vi "恢复参数.vi"(8 "仪器公式":T2(array[cluster]), 9 "量程参数":T3(array[cluster]), 10 "试剂容量参数":T4, 11 "外设参数":cluster{"仪器版本":T1, "error out":errorcluster}) -> (3 "恢复结果":string)   [LabVIEW 2016, in "斯坦道总磷总氮.lvlib"]
uses:
  <vilib>/NI/Progress Bar/Progress Bar.lvlib
  <vilib>/Utility/config.llb/NI_LVConfig.lvlib
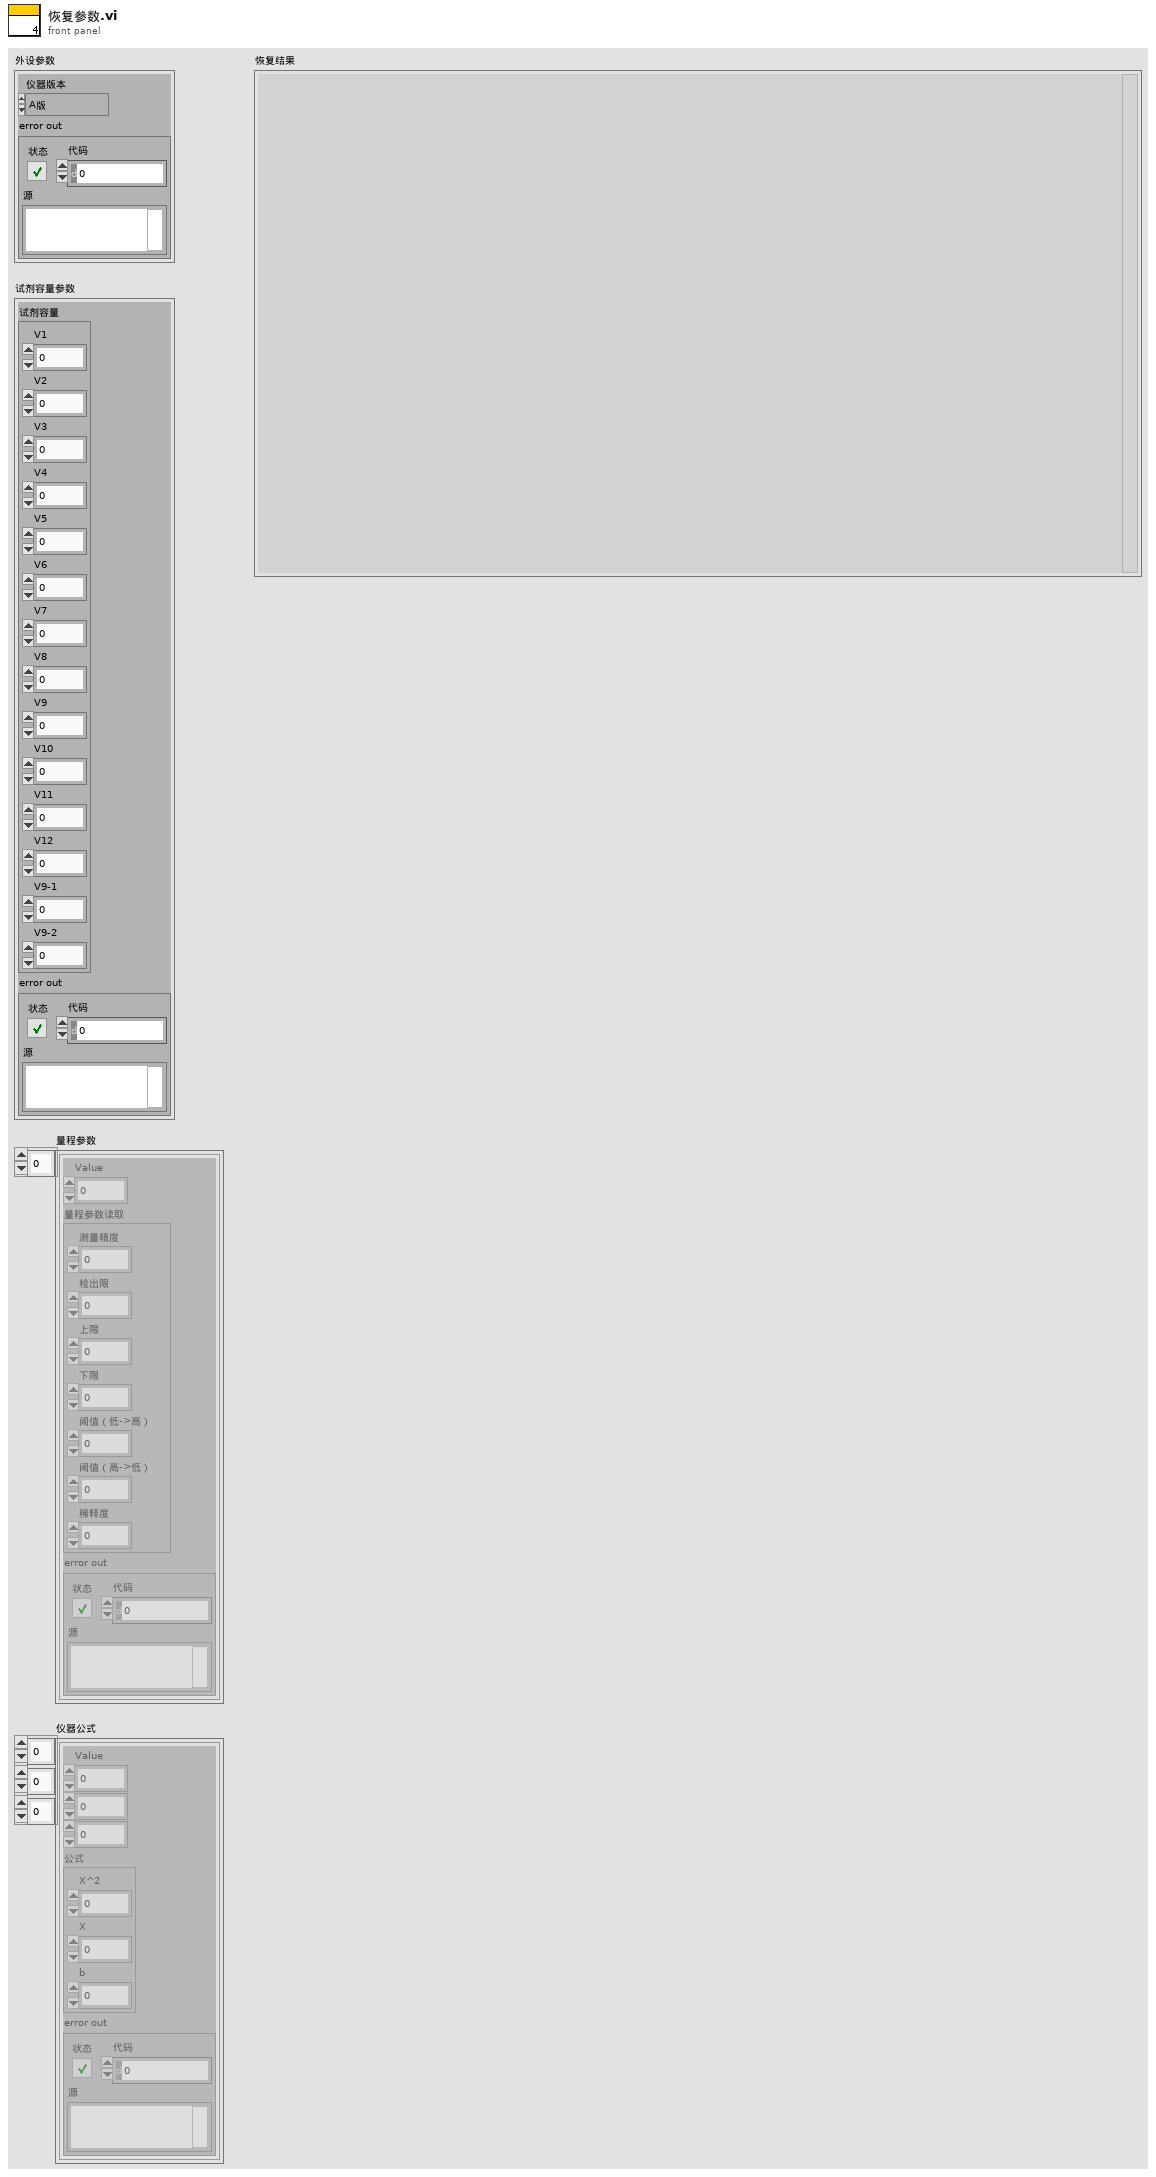
[diagram p1: front panel]
types:
  T1 = typedef "SingleStepTestV3.lvlib/SingleStepTestV3.lvclass/仪器版本.ctl" = enum16{"A版", "B版", "A1版"}
  T2 = cluster{"Value":u16, i32, i32, "公式":cluster{"X^2":dbl, "X":dbl, "b":dbl}, "error out":errorcluster}[][][]
  T3 = cluster{"Value":u16, "量程参数读取":cluster{"测量精度":u16, "检出限":dbl, "上限":dbl, "下限":dbl, "阈值（低->高）":dbl, "阈值（高->低）":dbl, "稀释度":dbl}, "error out":errorcluster}[]
  T4 = cluster{"试剂容量":cluster{"V1":sgl, "V2":sgl, "V3":sgl, "V4":sgl, "V5":sgl, "V6":sgl, "V7":sgl, "V8":sgl, "V9":sgl, "V10":sgl, "V11":sgl, "V12":sgl, "V9-1":sgl, "V9-2":sgl}, "error out":errorcluster}
  T5 = enum16{"恢复外设参数", "恢复试剂容量参数", "恢复量程参数", "恢复仪器公式", "结束"}
  T6 = typedef "NI_LVConfig.lvlib/Config Data RefNum.ctl" = refnum<k1>
  T7 = typedef "斯坦道总磷总氮.lvlib/V3 A版外设参数.ctl" = cluster{"泵类型":u8, "进样速度":u32, "出样速度":u32, "泵阀量":u8, "阀方向":u8, "光谱仪类型":u8, "光谱采样次数":u8, "氙灯次数":u8, "B":u16, "C":u16, "D":u16, "E":u16, "B_COD":u16, "C_COD":u16, "D_COD":u16, "E_COD":u16, "G":u16, "M":u16, "N":u16, "氨氮注射泵控温下限":sgl, "氨氮注射泵控温上限":sgl, "总氮注射泵控温下限":sgl, "总氮注射泵控温上限":sgl, "消解温度下限":sgl, "消解温度上限":sgl, "加热10s限值":sgl, "KP":sgl, "KI":sgl, "KD":sgl, "高温高压阀开阀温度":sgl, "总氮x公式0":u8, "总氮x公式1":sgl, "总氮x公式2":sgl, "总磷浊度稀释系数":sgl, "总磷浊度补偿权重1":sgl, "总磷浊度补偿权重2":sgl, "盐度系数":sgl, "氨氮补偿系数1":sgl, "氨氮补偿系数2":sgl}
  T8 = typedef "斯坦道总磷总氮.lvlib/V3 B版外设参数.ctl" = cluster{"泵类型":u8, "注射泵正常速度":u32, "注射泵慢速":u32, "阀型号":u8, "res":u8, "光谱仪类型":u8, "光谱采样次数":u8, "氙灯次数":u8, "B":u16, "C":u16, "D":u16, "E":u16, "B_COD":u16, "C_COD":u16, "D_COD":u16, "E_COD":u16, "G":u16, "M":u16, "N":u16, "降温下限":sgl, "降温上限":sgl, "恒温温度下限":sgl, "恒温温度上限":sgl, "消解温度下限":sgl, "消解温度上限":sgl, "加热10s限值":sgl, "KP":sgl, "KI":sgl, "KD":sgl, "高温高压阀开阀温度":sgl, "总氮x公式0":u8, "总氮x公式1":sgl, "总氮x公式2":sgl, "总磷浊度稀释系数":sgl, "总磷浊度补偿权重1":sgl, "总磷浊度补偿权重2":sgl, "盐度系数":sgl, "氨氮补偿系数1":sgl, "氨氮补偿系数2":sgl, "缺试剂传感器阈值":u16}
  T9 = typedef "斯坦道总磷总氮.lvlib/V3 A1版外设参数.ctl" = cluster{"泵类型":u8, "进样速度":u32, "出样速度":u32, "泵阀量":u8, "光谱仪类型":u8, "光谱采样次数":u8, "氙灯次数":u8, "B":u16, "C":u16, "D":u16, "E":u16, "B_COD":u16, "C_COD":u16, "D_COD":u16, "E_COD":u16, "G":u16, "M":u16, "N":u16, "氨氮注射泵控温下限":sgl, "氨氮注射泵控温上限":sgl, "总氮注射泵控温下限":sgl, "总氮注射泵控温上限":sgl, "消解温度下限":sgl, "消解温度上限":sgl, "加热10s限值":sgl, "高温高压阀开阀温度":sgl, "总氮x公式0":u8, "总氮x公式1":sgl, "总氮x公式2":sgl, "总磷浊度稀释系数":sgl, "总磷浊度补偿权重1":sgl, "总磷浊度补偿权重2":sgl, "盐度系数":sgl, "氨氮补偿系数1":sgl, "氨氮补偿系数2":sgl}
  T10 = cluster{"V1":sgl, "V2":sgl, "V3":sgl, "V4":sgl, "V5":sgl, "V6":sgl, "V7":sgl, "V8":sgl, "V9":sgl, "V10":sgl, "V11":sgl, "V12":sgl, "V9-1":sgl, "V9-2":sgl}
  T11 = cluster{"测量精度":u16, "检出限":dbl, "上限":dbl, "下限":dbl, "阈值（低->高）":dbl, "阈值（高->低）":dbl, "稀释度":dbl}
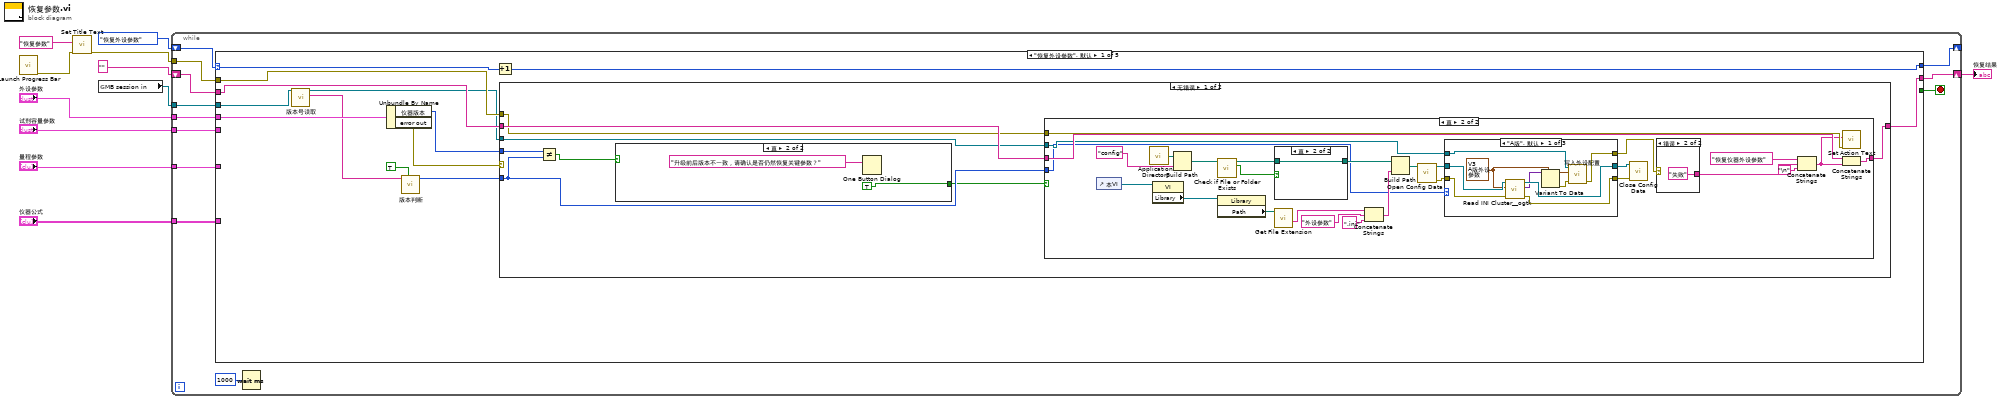
[diagram p0: block diagram]
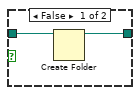
[diagram p3: hidden frame]
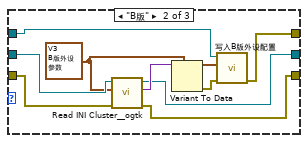
[diagram p4: hidden frame]
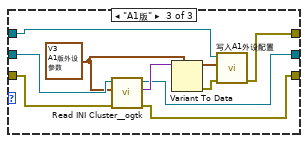
[diagram p5: hidden frame]
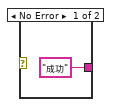
[diagram p6: hidden frame]
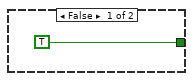
[diagram p7: hidden frame]
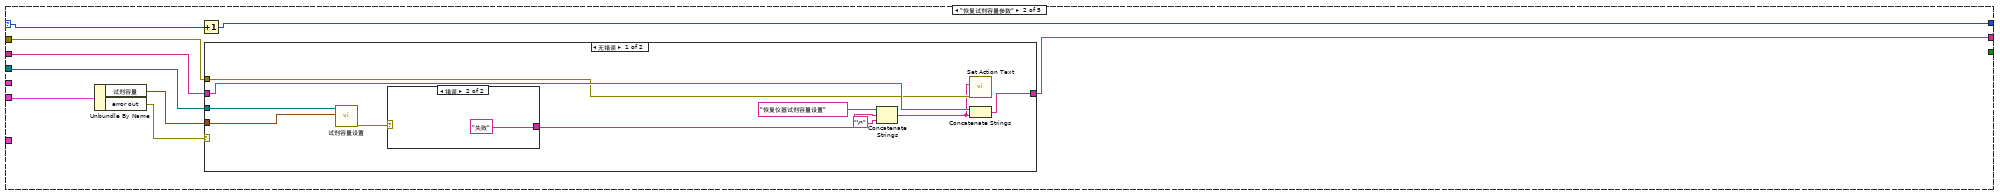
[diagram p9: hidden frame]
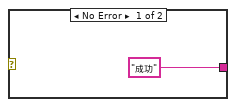
[diagram p10: hidden frame]
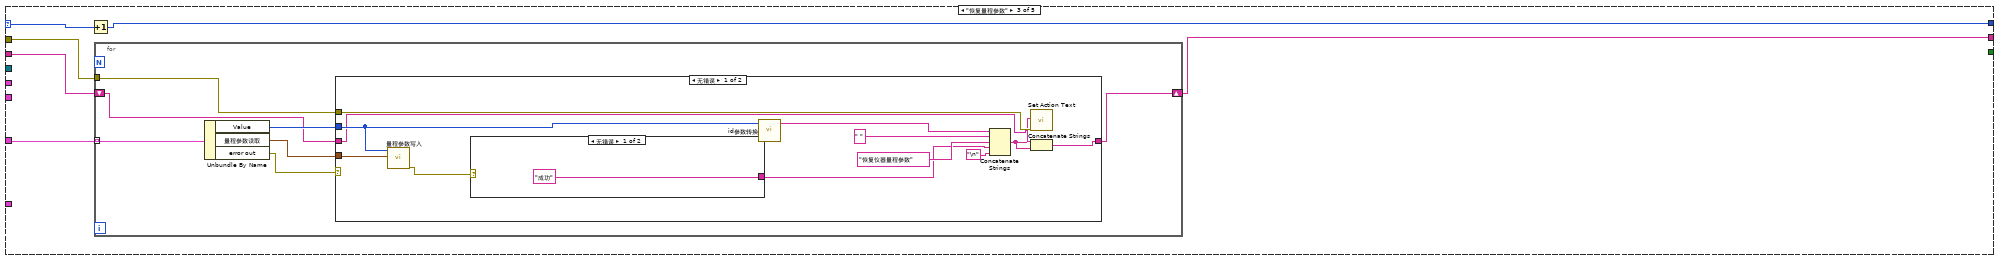
[diagram p12: hidden frame]
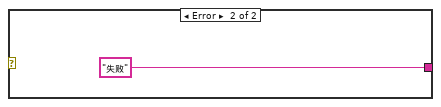
[diagram p13: hidden frame]
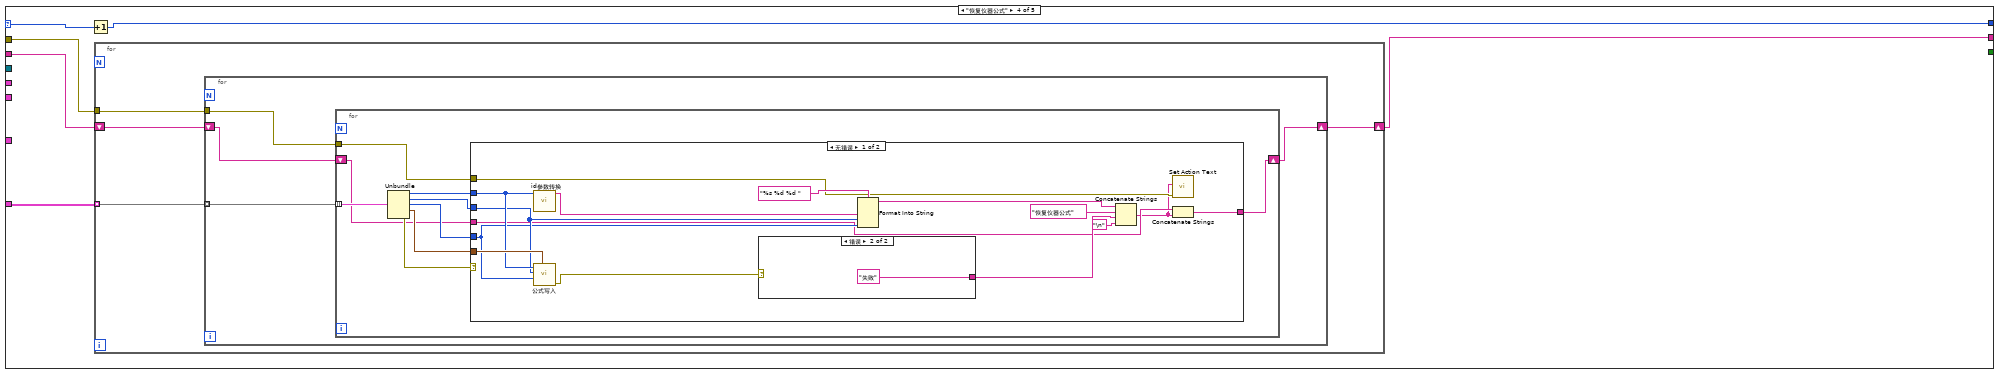
[diagram p15: hidden frame]
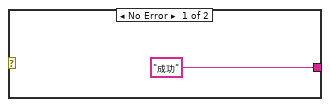
[diagram p16: hidden frame]
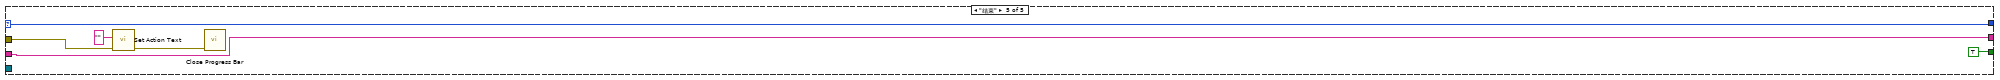
[diagram p18: hidden frame]
diagram:
  n1 = call <vilib>:"Launch Progress Bar.vi"() -> ("error out"=w4:errorcluster)  [unwired: 10 in, 1 out]
  n2 = call <vilib>:"Set Title Text.vi"("error in (no error)"=w4, "Installer Title"="恢复参数") -> ("error out"=w3:errorcluster)  [unwired: 9 in]
  n3 = global read "VAR总磷总氮全局变量.vi" "MB session in"() -> (w9:refnum<class "MB_Master.lvclass">)
  n4 = while {
    shift-right: [w22] -> _
    shift-left: T5."恢复外设参数" ("枚举") -> [w23]
    tunnel: "外设参数" -> [w21]
    shift-right: [w15] -> w5
    shift-left: "" -> [w20]
    tunnel: w9 -> [w19]
    tunnel: "试剂容量参数" -> [w18]
    tunnel: "量程参数" -> [w17]
    tunnel: "仪器公式" -> [w16]
    tunnel: w3 -> [w13]
    stop <- w14 stop-if-true
    n5 = case shown="\"恢复外设参数\", 默认" w23 {
      selector: w23 -> [w36 w121 w140 w168 w209]
      tunnel: [w35 w120 w139 w167 w209] -> w22
      tunnel: w21 -> [w30 _ _ _ _]
      tunnel: w20 -> [w33 w115 w137 w165 w208]
      tunnel: w19 -> [w28 w117 _ _ _]
      tunnel: w18 -> [_ w119 _ _ _]
      tunnel: w17 -> [_ _ w138 _ _]
      tunnel: w16 -> [_ _ _ w166 _]
      tunnel: [w32 w114 w136 w164 w208] -> w15
      tunnel: [_ _ _ _ TRUE] -> w14
      tunnel: w13 -> [w31 w113 w135 w163 w206]
      frame "恢复外设参数", Default {
        n6 = call "版本号读取.vi"("MB session in"=w28) -> ("固件版本号"=w26:string, "MB session out"=w27:refnum<class "MB_Master.lvclass">)  [unwired: 8 in, 1 out]
        n7 = Unbundle By Name(w30) -> ("仪器版本"=w24:T1, "error out"=w34:errorcluster)
        n8 = call "版本判断.vi"("Extern"=TRUE, "固件版本号"=w26) -> ("仪器版本"=w29:T1)  [unwired: 9 in]
        n9 = Increment(x=w36) -> (x+1=w35:T5)
        n10 = case shown="无错误" w34 {
          tunnel: w27 -> [w41 _]
          tunnel: w29 -> [w39 _]
          tunnel: [w43 w112] -> w32
          tunnel: w33 -> [w44 w112]
          tunnel: w31 -> [w42 _]
          tunnel: w24 -> [w40 _]
          frame No Error {
            n11 = Not Equal?(x=w40, y=w39) -> (x != y?=w38:bool)
            n12 = case shown="真" w38 {
              tunnel: [TRUE ("T button?") TRUE ("T button?")] -> w37
              frame False {
              }
              frame True {
                n13 = One Button Dialog(message="升级前后版本不一致，请确认是否仍然恢复关键参数？" ("消息")) -> ()  [unwired: 1 in, 1 out]
              }
            }
            n14 = case shown="真" w37 {
              tunnel: w44 -> [w45 w70]
              tunnel: [w45 w69] -> w43
              tunnel: w42 -> [_ w68]
              tunnel: w41 -> [_ w65]
              tunnel: w39 -> [_ w51]
              frame False {
              }
              frame True {
                n15 = control-ref of="本VI"() -> (w64:refnum<vi>)
                n16 = call <vilib>:"Application Directory.vi"() -> ("Application Directory"=w54:path)
                n17 = property class="VI"(reference=w64) -> ("Library"=w52:refnum<vi>)  [unwired: 1 in, 2 out]
                n18 = Build Path(base path=w54, name or relative path="config" ("名称或相对路径")) -> (appended path=w56:path)
                n19 = call <vilib>:"Check if File or Folder Exists.vi"("path"=w56) -> ("file or folder exists?"=w59:bool, "dup path"=w60:path)  [unwired: 8 in, 1 out]
                n20 = property class="Library"(reference=w52) -> ("Path"=w53:path)  [unwired: 1 in, 2 out]
                n21 = case shown="真" w59 {
                  tunnel: w60 -> [w75 w76]
                  tunnel: [w74 w76] -> w61
                  frame False {
                    n22 = Create Folder(path (use dialog)=w75) -> (created path=w74:path)  [unwired: 2 in, 2 out]
                  }
                  frame True {
                  }
                }
                n23 = call <vilib>:"Get File Extension.vi"("file"=w53) -> ("filename without extension"=w62:string)  [unwired: 6 in, 4 out]
                n24 = Concatenate Strings(w62, "外设参数" ("字符串"), ".ini" ("字符串")) -> (w58:string)
                n25 = Build Path(base path=w61, name or relative path=w58) -> (appended path=w50:path)
                n26 = call <vilib>:"Open Config Data.vi"("configuration file path"=w50) -> ("error out"=w48:errorcluster, "refnum"=w49:T6)  [unwired: 8 in, 1 out]
                n27 = case shown="\"A版\", 默认" w51 {
                  tunnel: [w86 w95 w105] -> w66
                  tunnel: w65 -> [w85 w96 w106]
                  tunnel: w49 -> [w84 w93 w103]
                  tunnel: w48 -> [w83 w92 w102]
                  tunnel: [w82 w90 w100] -> w47
                  tunnel: [w81 w91 w101] -> w46
                  frame "A版", Default {
                    w77 = T7 {"泵类型"=0, "进样速度"=0, "出样速度"=0, "泵阀量"=0, "阀方向"=0, "光谱仪类型"=0, "光谱采样次数"=0, "氙灯次数"=0, "B"=0, "C"=0, "D"=0, "E"=0, "B_COD"=0, "C_COD"=0, "D_COD"=0, "E_COD"=0, "G"=0, "M"=0, "N"=0, "氨氮注射泵控温下限"=0.0, "氨氮注射泵控温上限"=0.0, "总氮注射泵控温下限"=0.0, "总氮注射泵控温上限"=0.0, "消解温度下限"=0.0, "消解温度上限"=0.0, "加热10s限值"=0.0, "KP"=52.0, "KI"=1.156, "KD"=800.0, "高温高压阀开阀温度"=0.0, "总氮x公式0"=0, "总氮x公式1"=0.0, "总氮x公式2"=0.0, "总磷浊度稀释系数"=0.0, "总磷浊度补偿权重1"=0.0, "总磷浊度补偿权重2"=0.0, "盐度系数"=0.0, "氨氮补偿系数1"=0.0, "氨氮补偿系数2"=0.0} ("外设配置")
                    n28 = call <userlib>:"Read INI Cluster__ogtk.vi"("error in (no error)"=w83, "INI Fomatted Cluster Type"=w77, "refnum"=w84) -> ("error out"=w82:errorcluster, "INI Fomatted Cluster"=w80:variant, "dup refnum"=w81:T6)  [unwired: 4 in, 2 out]
                    n29 = Variant To Data(type=w77, Variant=w80) -> (data=w79:T7, error out=w78:errorcluster)  [unwired: 1 in]
                    n30 = call "写入外设配置.vi"("error in (no error)"=w78, "外设配置"=w79, "MB session in"=w85) -> ("error out"=w86:errorcluster)  [unwired: 7 in, 1 out]
                  }
                  frame "B版" {
                    w87 = T8 {"泵类型"=0, "注射泵正常速度"=0, "注射泵慢速"=0, "阀型号"=0, "res"=0, "光谱仪类型"=0, "光谱采样次数"=0, "氙灯次数"=0, "B"=0, "C"=0, "D"=0, "E"=0, "B_COD"=0, "C_COD"=0, "D_COD"=0, "E_COD"=0, "G"=0, "M"=0, "N"=0, "降温下限"=0.0, "降温上限"=0.0, "恒温温度下限"=0.0, "恒温温度上限"=0.0, "消解温度下限"=0.0, "消解温度上限"=0.0, "加热10s限值"=0.0, "KP"=0.0, "KI"=0.0, "KD"=0.0, "高温高压阀开阀温度"=0.0, "总氮x公式0"=0, "总氮x公式1"=0.0, "总氮x公式2"=0.0, "总磷浊度稀释系数"=0.0, "总磷浊度补偿权重1"=0.0, "总磷浊度补偿权重2"=0.0, "盐度系数"=0.0, "氨氮补偿系数1"=0.0, "氨氮补偿系数2"=0.0, "缺试剂传感器阈值"=0} ("外设配置")
                    n31 = call <userlib>:"Read INI Cluster__ogtk.vi"("error in (no error)"=w92, "INI Fomatted Cluster Type"=w87, "refnum"=w93) -> ("error out"=w90:errorcluster, "INI Fomatted Cluster"=w94:variant, "dup refnum"=w91:T6)  [unwired: 4 in, 2 out]
                    n32 = Variant To Data(type=w87, Variant=w94) -> (data=w89:T8, error out=w88:errorcluster)  [unwired: 1 in]
                    n33 = call "写入B版外设配置.vi"("error in (no error)"=w88, "外设配置"=w89, "MB session in"=w96) -> ("error out"=w95:errorcluster)  [unwired: 7 in, 1 out]
                  }
                  frame "A1版" {
                    w97 = T9 {"泵类型"=0, "进样速度"=0, "出样速度"=0, "泵阀量"=0, "光谱仪类型"=0, "光谱采样次数"=0, "氙灯次数"=0, "B"=0, "C"=0, "D"=0, "E"=0, "B_COD"=0, "C_COD"=0, "D_COD"=0, "E_COD"=0, "G"=0, "M"=0, "N"=0, "氨氮注射泵控温下限"=0.0, "氨氮注射泵控温上限"=0.0, "总氮注射泵控温下限"=0.0, "总氮注射泵控温上限"=0.0, "消解温度下限"=0.0, "消解温度上限"=0.0, "加热10s限值"=0.0, "高温高压阀开阀温度"=0.0, "总氮x公式0"=0, "总氮x公式1"=0.0, "总氮x公式2"=0.0, "总磷浊度稀释系数"=0.0, "总磷浊度补偿权重1"=0.0, "总磷浊度补偿权重2"=0.0, "盐度系数"=0.0, "氨氮补偿系数1"=0.0, "氨氮补偿系数2"=0.0} ("外设配置")
                    n34 = call <userlib>:"Read INI Cluster__ogtk.vi"("error in (no error)"=w102, "INI Fomatted Cluster Type"=w97, "refnum"=w103) -> ("error out"=w100:errorcluster, "INI Fomatted Cluster"=w104:variant, "dup refnum"=w101:T6)  [unwired: 4 in, 2 out]
                    n35 = Variant To Data(type=w97, Variant=w104) -> (data=w99:T9, error out=w98:errorcluster)  [unwired: 1 in]
                    n36 = call "写入A1外设配置.vi"("error in (no error)"=w98, "外设配置"=w99, "MB session in"=w106) -> ("error out"=w105:errorcluster)  [unwired: 7 in, 1 out]
                  }
                }
                n37 = call <vilib>:"Close Config Data.vi"("error in (no error)"=w47, "refnum"=w46) -> ()  [unwired: 8 in, 2 out]
                n38 = case shown="错误" w66 {
                  tunnel: ["成功" "失败"] -> w72
                  frame No Error {
                  }
                  frame Error {
                  }
                }
                n39 = Concatenate Strings("恢复仪器外设参数" ("字符串"), w72, "\n") -> (w67:string)
                n40 = call <vilib>:"Set Action Text.vi"("error in (no error)"=w68, "Action Text"=w67) -> ()  [unwired: 9 in, 1 out]
                n41 = Concatenate Strings(w70, w67) -> (w69:string)
              }
            }
          }
          frame Error {
          }
        }
      }
      frame "恢复试剂容量参数" {
        n42 = Unbundle By Name(w119) -> ("试剂容量"=w118:T10, "error out"=w116:errorcluster)
        n43 = Increment(x=w121) -> (x+1=w120:T5)
        n44 = case shown="无错误" w116 {
          tunnel: w118 -> [w131 _]
          tunnel: w117 -> [w130 _]
          tunnel: w115 -> [w125 w134]
          tunnel: [w124 w134] -> w114
          tunnel: w113 -> [w123 _]
          frame No Error {
            n45 = call "试剂容量设置.vi"("试剂容量"=w131, "MB session in"=w130) -> ("error out"=w127:errorcluster)  [unwired: 8 in, 1 out]
            n46 = case shown="错误" w127 {
              tunnel: ["成功" "失败"] -> w128
              frame No Error {
              }
              frame Error {
              }
            }
            n47 = Concatenate Strings("恢复仪器试剂容量设置" ("字符串"), w128, "\n") -> (w122:string)
            n48 = call <vilib>:"Set Action Text.vi"("error in (no error)"=w123, "Action Text"=w122) -> ()  [unwired: 9 in, 1 out]
            n49 = Concatenate Strings(w125, w122) -> (w124:string)
          }
          frame Error {
          }
        }
      }
      frame "恢复量程参数" {
        n50 = Increment(x=w140) -> (x+1=w139:T5)
        n51 = for {
          tunnel: w138 -> [w147] mode=indexing
          shift-right: [w142] -> w136
          shift-left: w137 -> [w143]
          tunnel: w135 -> [w141]
          n52 = Unbundle By Name(w147) -> ("Value"=w145:u16, "量程参数读取"=w146:T11, "error out"=w144:errorcluster)
          n53 = case shown="无错误" w144 {
            tunnel: w146 -> [w159 _]
            tunnel: w145 -> [w155 _]
            tunnel: w143 -> [w151 w162]
            tunnel: [w150 w162] -> w142
            tunnel: w141 -> [w149 _]
            frame No Error {
              n54 = call "量程参数写入.vi"("量程参数写入"=w159, "测量参数"=w155) -> ("error out"=w156:errorcluster)  [unwired: 8 in]
              n55 = case shown="无错误" w156 {
                tunnel: ["成功" "失败"] -> w157
                frame No Error {
                }
                frame Error {
                }
              }
              n56 = call "id参数转换.vi"("id"=w155) -> ("table输出"=w154:string)  [unwired: 9 in, 1 out]
              n57 = Concatenate Strings(w154, " " ("字符串"), "恢复仪器量程参数" ("字符串"), w157, "\n") -> (w148:string)
              n58 = call <vilib>:"Set Action Text.vi"("error in (no error)"=w149, "Action Text"=w148) -> ()  [unwired: 9 in, 1 out]
              n59 = Concatenate Strings(w151, w148) -> (w150:string)
            }
            frame Error {
            }
          }
        }
      }
      frame "恢复仪器公式" {
        n60 = Increment(x=w168) -> (x+1=w167:T5)
        n61 = for {
          tunnel: w166 -> [w172] mode=indexing
          shift-right: [w170] -> w164
          shift-left: w165 -> [w171]
          tunnel: w163 -> [w169]
          n62 = for {
            tunnel: w172 -> [w176] mode=indexing
            shift-right: [w174] -> w170
            shift-left: w171 -> [w175]
            tunnel: w169 -> [w173]
            n63 = for {
              tunnel: w176 -> [w185] mode=indexing
              shift-right: [w178] -> w174
              shift-left: w175 -> [w179]
              tunnel: w173 -> [w177]
              n64 = Unbundle(w185) -> ("Value"=w183:u16, w182:i32, w181:i32, "公式"=w180:cluster{"X^2":dbl, "X":dbl, "b":dbl}, "error out"=w184:errorcluster)
              n65 = case shown="无错误" w184 {
                tunnel: w183 -> [w193 _]
                tunnel: w182 -> [w192 _]
                tunnel: w181 -> [w191 _]
                tunnel: w180 -> [w200 _]
                tunnel: w179 -> [w189 w203]
                tunnel: [w188 w203] -> w178
                tunnel: w177 -> [w187 _]
                frame No Error {
                  n66 = call "id参数转换.vi"("id"=w193) -> ("table输出"=w196:string)  [unwired: 9 in, 1 out]
                  n67 = call "公式写入.vi"("公式"=w200, "量程"=w191, "测量模式"=w192, "测量参数"=w193) -> ("error out"=w194:errorcluster)  [unwired: 7 in]
                  n68 = case shown="错误" w194 {
                    tunnel: ["成功" "失败"] -> w199
                    frame No Error {
                    }
                    frame Error {
                    }
                  }
                  n69 = Format Into String(format string="%s %d %d " ("格式字符串"), w196, w192, w191) -> (resulting string=w195:string)  [unwired: 2 in, 1 out]
                  n70 = Concatenate Strings(w195, "恢复仪器公式" ("字符串"), w199, "\n") -> (w186:string)
                  n71 = call <vilib>:"Set Action Text.vi"("error in (no error)"=w187, "Action Text"=w186) -> ()  [unwired: 9 in, 1 out]
                  n72 = Concatenate Strings(w189, w186) -> (w188:string)
                }
                frame Error {
                }
              }
            }
          }
        }
      }
      frame "结束" {
        n73 = call <vilib>:"Set Action Text.vi"("error in (no error)"=w206, "Action Text"="") -> ("error out"=w205:errorcluster)  [unwired: 9 in]
        n74 = call <vilib>:"Close Progress Bar.vi"("error in (no error)"=w205) -> ()  [unwired: 9 in, 2 out]
      }
    }
    n75 = Wait (ms)(milliseconds to wait=u32 1000 ("等待时间（毫秒）")) -> ()  [unwired: 1 out]
  }
  "恢复结果" <- w5
